vi "Error Log Ref (library variable).vi"() -> ()   [LabVIEW 2023, in "Error Manager.lvlib" / "Error Log.lvclass"]
uses:
  Error Log.lvclass
panel:
  in  "Error Log Ref":refnum<file>
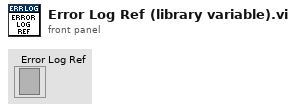
[diagram p1: front panel]
diagram:
